vi "To XML - Returns XML Entities.vi"() -> ()   [LabVIEW 2017, in "Cobertura.Tests.lvlib" / "Coverage.lvlib"]
uses:
  Coverage.lvlib
  <vilib>/xml/Close Reference(Node).vi
  Cobertura/Coverage/Coverage.lvclass
  <vilib>/xml/NI_XML.lvlib
  <resource>/objmgr/DOMUserDefRef.rc
  <vilib>/PNR/Transparent Assertions/Transparent Assertions/Transparent Assertions.lvlib
panel:
  out "error out":errorcluster
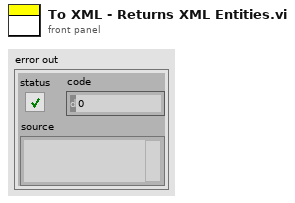
[diagram p1: front panel]
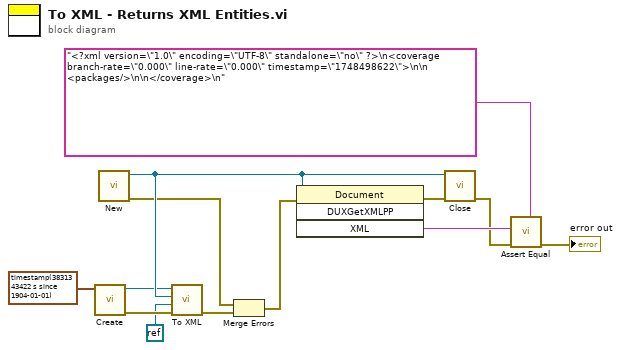
[diagram p0: block diagram]
diagram:
  n1 = call "Create.vi"("Timestamp"=timestamp(3831343422.3303647 s since 1904-01-01)) -> ("error out"=w13:errorcluster, "Coverage"=w4:refnum<class "Coverage.lvclass">)  [unwired: 9 in]
  n2 = call <vilib>:"New.vi"() -> ("error out"=w3:errorcluster, "DOM document out"=w11:refnum<k20>)  [unwired: 8 in]
  n3 = call-dynamic "To XML.vi"("error in (no error)"=w13, "Parent"=refnum<k0> refnum, "Document"=w11, "Coverage in"=w4) -> ("error out"=w6:errorcluster)  [unwired: 7 in]
  n4 = Merge Errors(w3, w6) -> (w7:errorcluster)
  n5 = invoke class="Document" method="DUXGetXMLPP"(reference=w11, error in=w7) -> (error out=w12:errorcluster, "XML"=w10:string)  [unwired: 2 in, 2 out]
  n6 = call-poly <vilib>:"Close.vi"("error in (no error)"=w12, "node"=w11) -> ("error out"=w2:errorcluster)  [unwired: 7 in]
  n7 = call <vilib>:"Assert Equal.vi"("Expected"="<?xml version=\"1.0\" encoding=\"UTF-8\" standalone=\"no\" ?>\n<coverage branch-rate=\"0.000\" line-rate=\"0.000\" timestamp=\"1748498622\">\n\n  <packages/>\n\n</coverage>\n", "error in (no error)"=w2, "Actual"=w10) -> ("error out"=→"error out":errorcluster)  [unwired: 8 in]
